vi "set_counter.vi"(8 "error in (no error)":errorcluster, 10 "counter":tag, 11 "SignalWriterDL090202DAQmx in":refnum<class "SignalWriterDL090202DAQmx.lvclass">) -> (0 "error out":errorcluster, 3 "SignalWriterDL090202DAQmx out":refnum<class "SignalWriterDL090202DAQmx.lvclass">)   [LabVIEW 2010, in "SignalWriterDL090202DAQmx.lvclass"]
uses:
  SignalWriterDL090202DAQmx.lvclass
  SignalWriterDL090202DAQmx.lvclass/SignalWriterDL090202DAQmx.ctl
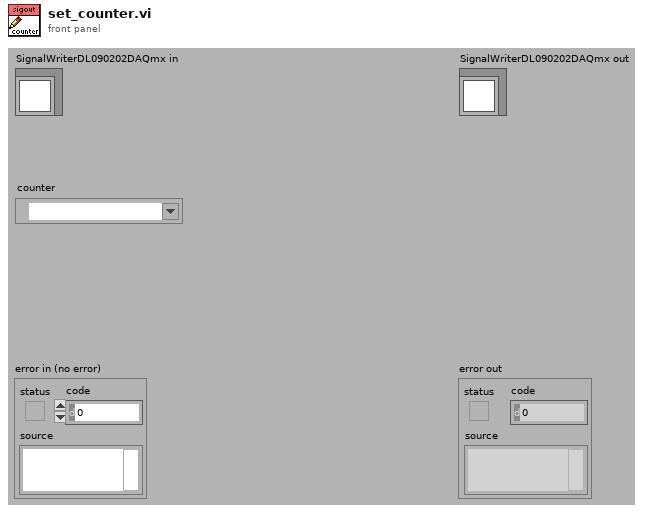
[diagram p1: front panel]
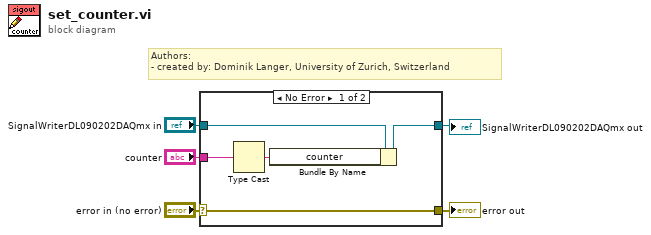
[diagram p0: block diagram]
diagram:
  # "Authors: \n- created by: Dominik Langer, University of Zurich, Switzerland"
  n1 = case shown="No Error" "error in (no error)" {
    selector: "error in (no error)" -> [w10 w12]
    tunnel: [w10 w12] -> w4
    tunnel: [w6 w11] -> w2
    tunnel: "SignalWriterDL090202DAQmx in" -> [w7 w11]
    tunnel: "counter" -> [w8 _]
    frame No Error {
      n2 = Type Cast(x=w8) -> (*(type *) &x=w9:string)  [unwired: 1 in]
      n3 = Bundle By Name(cluster=w7, "counter"=w9) -> (w6:refnum<class "SignalWriterDL090202DAQmx.lvclass">)
    }
    frame Error {
    }
  }
  "error out" <- w4
  "SignalWriterDL090202DAQmx out" <- w2
